vi "Find PeaksValleys.vi"(4 "peaks/valleys":enum32{"Peaks", "Valleys"}(ring), 6 "Options":T1, 8 "error in (no error)":errorcluster, 9 "Data Array":dbl[](array[numeric]), 10 "XYGraph in":refnum<vi>, 11 "input picture in":picture) -> (0 "error out":errorcluster, 2 "XYGraph out":refnum<vi>, 3 "input picture out":picture)   [LabVIEW 2014, in "Graph Extensions.lvlib"]
uses:
  Graph Extensions.lvlib
  <vilib>/Analysis/NI_AAL_SigProc.lvlib
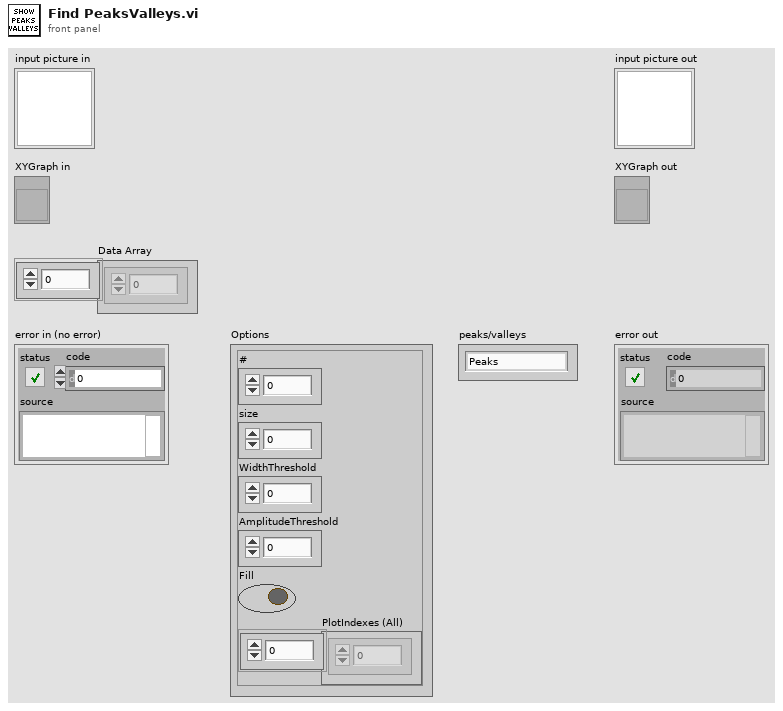
[diagram p1: front panel]
types:
  T1 = cluster{"#":i32, "size":i16, "WidthThreshold":i32, "AmplitudeThreshold":dbl, "Fill":bool, "PlotIndexes (All)":u16[]}
  T2 = typedef "LVRectTypeDef.ctl" = cluster{"Left":i16, "Top":i16, "Right":i16, "Bottom":i16}
  T3 = cluster{"Numeric Control":dbl, "Numeric Control":dbl}
  T4 = typedef "LVPoint32TypeDef.ctl" = cluster{"Horizontal":i32, "Vertical":i32}
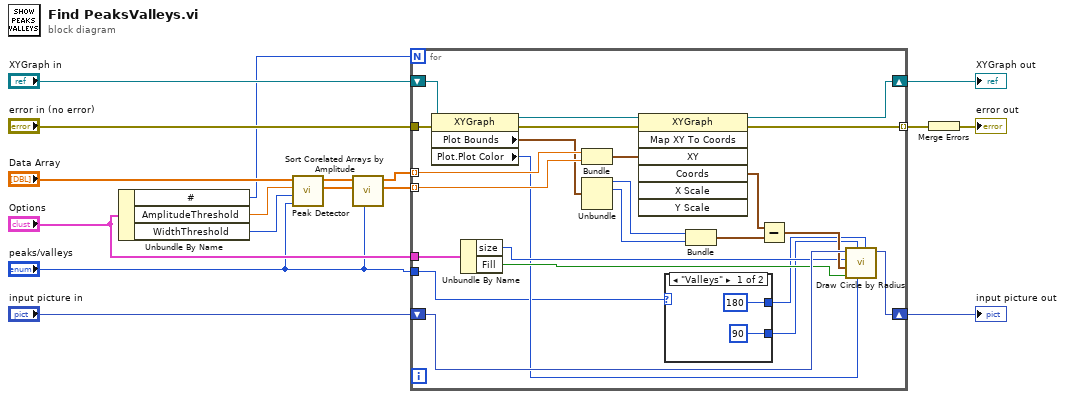
[diagram p0: block diagram]
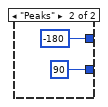
[diagram p2: hidden frame]
diagram:
  n1 = Unbundle By Name("Options") -> ("#"=w4:i32, "AmplitudeThreshold"=w16:dbl, "WidthThreshold"=w15:i32)
  n2 = call <vilib>:"Peak Detector.vi"("peaks/valleys"="peaks/valleys", "width"=w15, "threshold"=w16, "X"="Data Array") -> ("Amplitudes"=w11:dbl[], "Locations"=w10:dbl[])  [unwired: 3 in, 3 out]
  n3 = call "Sort Corelated Arrays by Amplitude.vi"("peaks/valleys"="peaks/valleys", "Amplitudes"=w11, "Locations"=w10) -> ("Amplitudes SORTED DESC"=w2:dbl[], "Locations Sorted"=w3:dbl[])  [unwired: 7 in]
  n4 = for {
    N: w4 -> [_]
    tunnel: "Options" -> [w31]
    tunnel: w3 -> [w41] mode=indexing
    tunnel: w2 -> [w40] mode=indexing
    shift-right: [w38] -> w13
    shift-left: "input picture in" -> [w39]
    shift-right: [w28] -> w6
    shift-left: "XYGraph in" -> [w27]
    tunnel: "error in (no error)" -> [w23]
    tunnel: [w21] -> w7 mode=indexing
    tunnel: "peaks/valleys" -> [w18]
    n5 = property class="XYGraph"(reference=w27, error in=w23) -> (reference out=w26:refnum<vi>, error out=w22:errorcluster, "Plot Bounds"=w24:T2, "Plot.Plot Color"=w25:u32)
    n6 = Unbundle By Name(w31) -> ("size"=w30:i16, "Fill"=w29:bool)
    n7 = Bundle("Numeric Control"=w41, "Numeric Control"=w40) -> (w37:T3)  [unwired: 1 in]
    n8 = Unbundle(w24) -> ("Left"=w35:i16, "Top"=w34:i16)  [unwired: 2 out]
    n9 = invoke on="Invoke Node" class="XYGraph" method="Map XY To Coords"(reference=w26, error in=w22, "XY"=w37) -> (reference out=w28:refnum<vi>, error out=w21:errorcluster, "Coords"=w33:T4)  [unwired: 4 in, 4 out]
    n10 = case shown="\"Valleys\"" w18 {
      tunnel: [i16 90 ("start angle(0)") i16 90 ("start angle(0)")] -> w20
      tunnel: [i16 180 ("start angle(0)") i16 -180 ("start angle(0)")] -> w19
      frame "Valleys" {
      }
      frame "Peaks" {
      }
    }
    n11 = Bundle("Left"=w35, "Top"=w34) -> (w36:cluster{"Left":i16, "Top":i16})  [unwired: 1 in]
    n12 = Subtract(x=w33, y=w36) -> (x-y=w32:T4)
    n13 = call <vilib>:"Draw Circle by Radius.vi"("arc size(360)"=w19, "color(black)"=w25, "start angle(0)"=w20, "fill?(F)"=w29, "pixel center"=w32, "radius"=w30, "picture"=w39) -> ("new picture"=w38:picture)  [unwired: 4 in]
  }
  "input picture out" <- w13
  "XYGraph out" <- w6
  n14 = Merge Errors(w7) -> (→"error out":errorcluster)
